vi "任务A.vi"(8 "error in (no error)":errorcluster caption="错误输入（无错误）", 10 "测试条目":i32) -> (0 "error out":errorcluster caption="错误输出", 2 "数值":dbl)   [LabVIEW 2022 SP3]
doc: "本VI是为《我和LabVIEW》一书编写的示例。\n关于本书的介绍请参考网页：\nhttp://ruanqizhen.spaces.live.com/blog/cns!5852D4F797C53FB6!4310.entry"
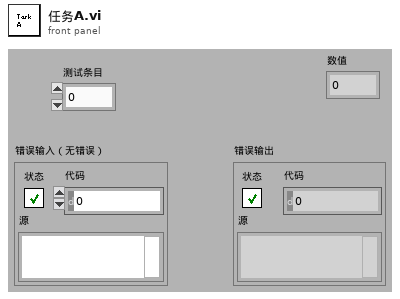
[diagram p1: front panel]
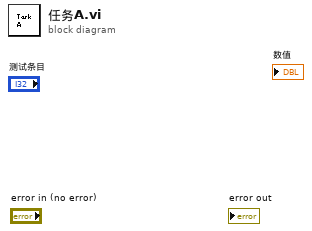
[diagram p0: block diagram]
diagram:
